vi "_save_csv.vi"(7 "delimiter (\\t)":string="SingleCh_", 11 "Data":dbl[][](array[numeric])) -> (3 "FileName":string)   [LabVIEW 2023]
uses:
  <vilib>/Utility/file.llb/Write Delimited Spreadsheet (string).vi
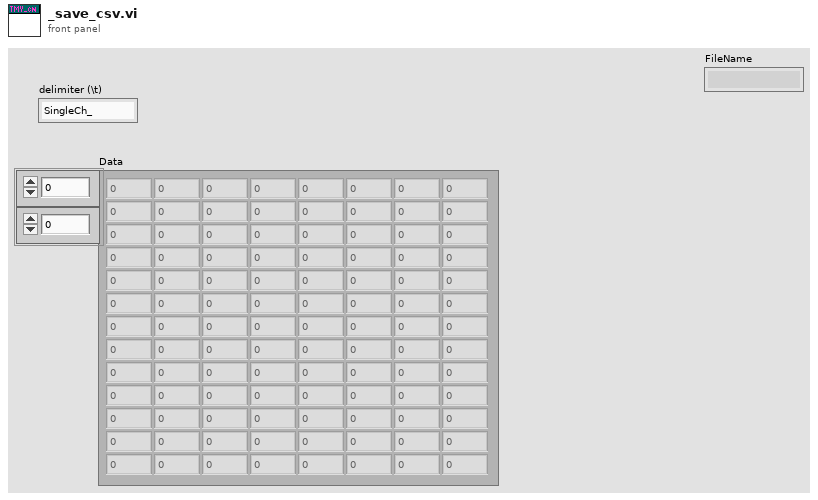
[diagram p1: front panel]
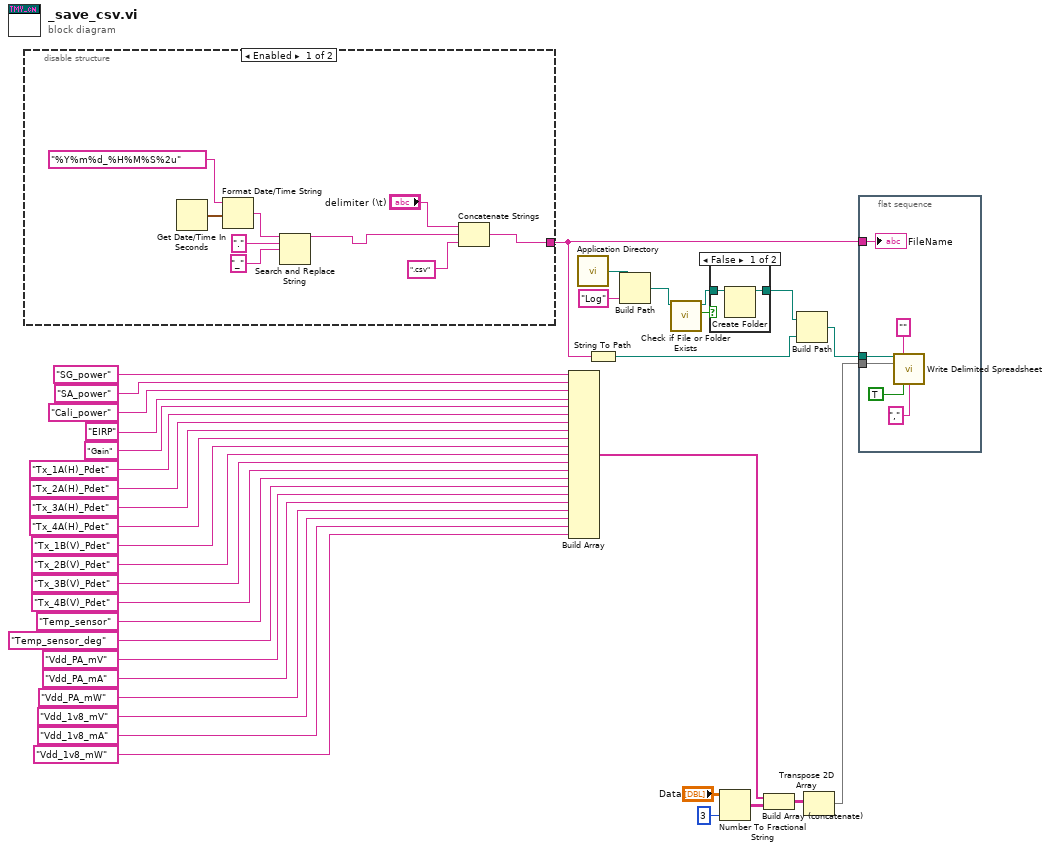
[diagram p0: block diagram]
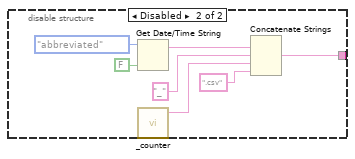
[diagram p3: hidden frame]
diagram:
  n1 = disable-structure shown="Enabled" {
    disable-tunnel: [w44 w46] -> w33
    frame Enabled {
      n2 = Get Date/Time In Seconds() -> (seconds since 1Jan1904=w42:timestamp)
      n3 = Format Date/Time String(time format string (%c)="%Y%m%d_%H%M%S%2u", seconds (now)=w42) -> (date/time string=w40:string)  [unwired: 1 in]
      n4 = Search and Replace String(input string=w40, search string=".", replace string="_") -> (result string=w37:string)  [unwired: 5 in, 3 out]
      n5 = Concatenate Strings("delimiter (\\t)", w37, ".csv" ("delimiter (\\t)")) -> (w44:string)
    }
    frame Disabled {
      n6 = Get Date/Time String(date format (0)=enum16{"short", "long", "abbreviated"}."abbreviated", want seconds? (F)=FALSE) -> (date string=w53:string)  [unwired: 1 in, 1 out]
      n7 = call "_counter.vi"() -> ("out_count"=w47:string)  [unwired: 5 in]
      n8 = Concatenate Strings(w53, "_" ("delimiter (\\t)"), w47, ".csv" ("delimiter (\\t)")) -> (w46:string, w48:string)
    }
  }
  n9 = Build Array("SG_power", "SA_power", "Cali_power", "EIRP", "Gain", "Tx_1A(H)_Pdet", "Tx_2A(H)_Pdet", "Tx_3A(H)_Pdet", "Tx_4A(H)_Pdet", "Tx_1B(V)_Pdet", "Tx_2B(V)_Pdet", "Tx_3B(V)_Pdet", "Tx_4B(V)_Pdet", "Temp_sensor", "Temp_sensor_deg", "Vdd_PA_mV", "Vdd_PA_mA", "Vdd_PA_mW", "Vdd_1v8_mV", "Vdd_1v8_mA", "Vdd_1v8_mW") -> (w22:string[])
  n10 = call <vilib>:"Application Directory.vi"() -> ("Application Directory"=w32:path)
  n11 = String To Path(string=w33) -> (path=w35:path)
  n12 = Build Path(base path=w32, name or relative path="Log") -> (appended path=w29:path)
  n13 = call <vilib>:"Check if File or Folder Exists.vi"("path"=w29) -> ("file or folder exists?"=w31:bool, "dup path"=w30:path)  [unwired: 8 in, 1 out]
  n14 = case shown="False" w31 {
    tunnel: w30 -> [w55 w56]
    tunnel: [w54 w56] -> w28
    frame False {
      n15 = Create Folder(path (use dialog)=w55) -> (created path=w54:path)  [unwired: 2 in, 2 out]
    }
    frame True {
    }
  }
  n16 = Number To Fractional String(number="Data", precision (6)=i16 3) -> (F-format string=w23:string[][])  [unwired: 2 in]
  n17 = Build Array (concatenate)(w22, w23) -> (w21:string[][])
  n18 = Build Path(base path=w28, name or relative path=w35) -> (appended path=w34:path)
  n19 = Transpose 2D Array(2D array=w21) -> (transposed array=w20:string[][])
  n20 = flat-sequence {
    tunnel: w34 -> [w61]
    tunnel: w33 -> [w59]
    tunnel: w20 -> [w57]
    frame #0 {
      n21 = call-poly <vilib>:"Write Delimited Spreadsheet.vi"("file path (dialog if empty)"=w61, "format (%s)"="" ("format (%.3f)"), "2D data"=w57, "transpose? (no:F)"=TRUE, "delimiter (\\t)"="," ("delimiter (\\t)")) -> ()  [unwired: 9 in, 2 out]
      "FileName" <- w59
    }
  }
